vi "UniCyRO Environment Simulator.vi"() -> ()   [LabVIEW 2012]
doc: "This VI starts and stops the environment simulator and serves as the master VI for your simulation code. Open and run this VI to display the environment simulator, or open the block diagram to view or modify simulation code."
uses:
  <vilib>/robotics/Simulator/Engine/ctl/DeviceID.ctl
  <instrlib>/Sparkfun Atomic IMU/HAIOL/Sparkfun Atomic IMU.lvclass
  <vilib>/robotics/Simulator/NI_Robotics_Simulator.lvlib
  <instrlib>/Sparkfun Atomic IMU/HAIOL/Simulator/Sparkfun Atomic IMU Simulator.lvclass
panel:
  in  "Device ID":T1
  in  "manifest filename":string="UniCyRO Environment Simulator.xml"
  in  "stop":bool
  # "* Press the Run button to display the Robotics Environment Simulator.\n* Select Window>>Show Block Diagram or press <Ctrl-E> to view the block diagram, where you can add or modify simulation code. Add controls and indicators to the front panel of this VI to pass data into and out of the simulation code.\n* The manifest file must exist in same directory as the .lvproj file."
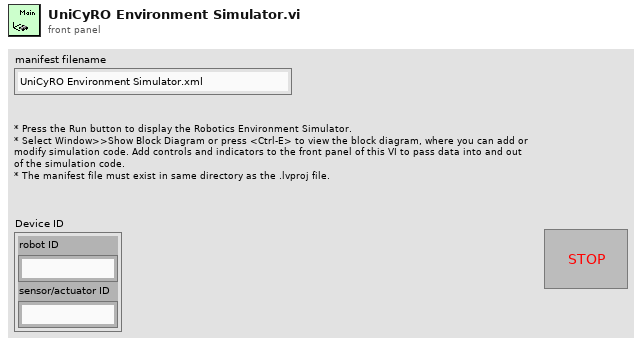
[diagram p1: front panel]
types:
  T1 = typedef "NI_Robotics_Simulator.lvlib/DeviceID.ctl" = cluster{"robot ID":string, "sensor/actuator ID":string}
  T2 = enum8{"50Hz", "100Hz", "150Hz", "200Hz", "250Hz"}
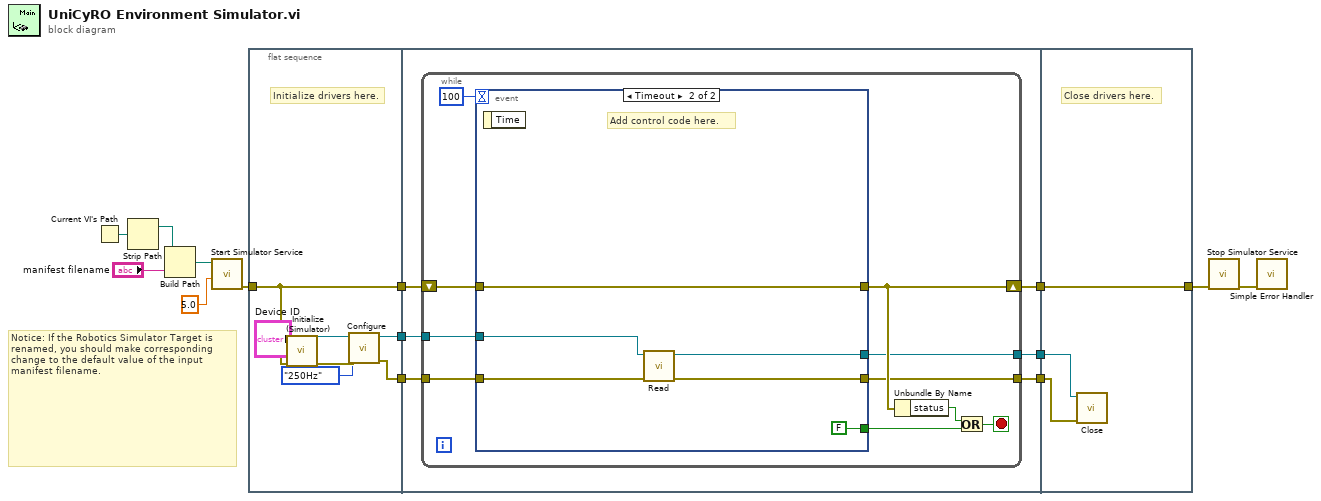
[diagram p0: block diagram]
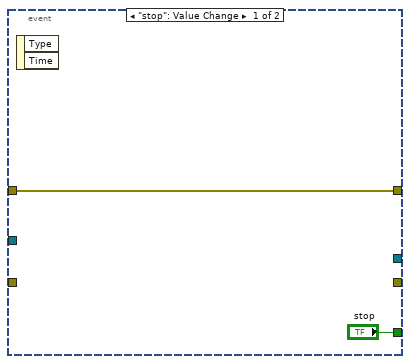
[diagram p2: hidden frame]
diagram:
  # "Notice: If the Robotics Simulator Target is renamed, you should make corresponding change to the default value of the input manifest filename."
  n1 = Current VI's Path() -> (path=w12:path)
  n2 = Strip Path(path=w12) -> (stripped path=w11:path)  [unwired: 1 out]
  n3 = Build Path(base path=w11, name or relative path="manifest filename") -> (appended path=w10:path)
  n4 = call <vilib>:"Start Simulator Service.vi"("step size (ms)"=5.0 ("stepsize(ms)"), "manifest file"=w10) -> ("error out"=w7:errorcluster)  [unwired: 9 in]
  n5 = flat-sequence {
    tunnel: w7 -> [w16]
    tunnel: [w16] -> w6
    tunnel: [w20] -> w4
    tunnel: [w19] -> w1
    tunnel: w6 -> [w26]
    tunnel: [w27] -> w5
    tunnel: w4 -> [w25]
    tunnel: [w24] -> w3
    tunnel: [w23] -> w2
    tunnel: w1 -> [w22]
    tunnel: [w48] -> w13
    tunnel: w5 -> [w48]
    tunnel: w3 -> [w47]
    tunnel: w2 -> [w46]
    frame #0 {
      # "Initialize drivers here."
      n6 = call <instrlib>:"Initialize (Simulator).vi"("error in (no error)"=w16, "Device ID"="Device ID") -> ("error out"=w21:errorcluster, "Sparkfun Atomic IMU out"=w18:refnum<class "Sparkfun Atomic IMU.lvclass">)  [unwired: 8 in]
      n7 = call-dynamic "Configure.vi"("error in (no error)"=w21, "Sample Frequency (100Hz)"=T2."250Hz", "Sparkfun Atomic IMU in"=w18) -> ("error out"=w20:errorcluster, "Sparkfun Atomic IMU out"=w19:refnum<class "Sparkfun Atomic IMU.lvclass">)  [unwired: 7 in]
    }
    frame #1 {
      n8 = while {
        shift-right: [w33] -> w27
        shift-left: w26 -> [w36]
        tunnel: w25 -> [w31]
        tunnel: [w30] -> w24
        tunnel: [w29] -> w23
        tunnel: w22 -> [w28]
        stop <- w34 stop-if-true
        n9 = event shown="[1] Timeout" {
          selector: _ -> [_ _]
          dyn-events: _ -> [_ _]
          timeout: 100 -> [_ _]
          tunnel: ["stop" FALSE ("stop")] -> w35
          tunnel: [w38 w45] -> w33
          tunnel: w36 -> [w38 w45]
          tunnel: w31 -> [_ w43]
          tunnel: [_ w42] -> w30
          tunnel: [_ w41] -> w29
          tunnel: w28 -> [_ w40]
          event "stop": Value Change {
            n10 = event-data() -> ()  [unwired: 1 in, 2 out]
          }
          event Timeout {
            # "Add control code here."
            n11 = event-data() -> ()  [unwired: 1 in, 1 out]
            n12 = call-dynamic "Read.vi"("error in (no error)"=w43, "Sparkfun Atomic IMU in"=w40) -> ("error out"=w42:errorcluster, "Sparkfun Atomic IMU out"=w41:refnum<class "Sparkfun Atomic IMU.lvclass">)  [unwired: 6 in, 2 out]
          }
        }
        n13 = Unbundle By Name(w33) -> ("status"=w32:bool)
        n14 = Or(x=w32, y=w35) -> (x .or. y?=w34:bool)
      }
    }
    frame #2 {
      # "Close drivers here."
      n15 = call-dynamic "Close.vi"("error in (no error)"=w47, "Sparkfun Atomic IMU in"=w46) -> ()  [unwired: 9 in, 1 out]
    }
  }
  n16 = call <vilib>:"Stop Simulator Service.vi"("error in (no error)"=w13) -> ("error out"=w8:errorcluster)  [unwired: 10 in]
  n17 = call <vilib>:"Simple Error Handler.vi"("error in (no error)"=w8) -> ()  [unwired: 4 in, 5 out]
